vi "GetEventHardpointMonitorWarningField.vi"(10 "Event Data":string, 11 "Cluster in":refnum<vi>) -> (3 "Array":string[](array[string]))   [LabVIEW 2016]
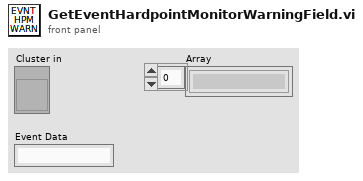
[diagram p1: front panel]
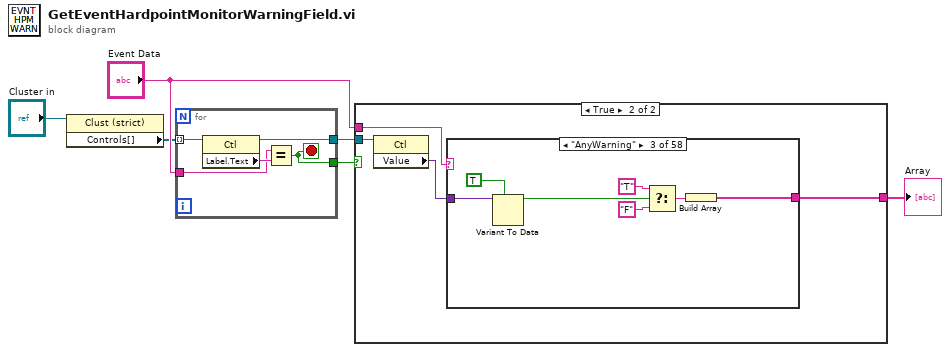
[diagram p0: block diagram]
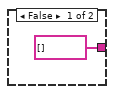
[diagram p2: hidden frame]
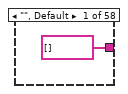
[diagram p3: hidden frame]
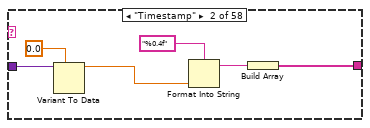
[diagram p4: hidden frame]
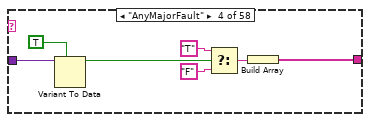
[diagram p5: hidden frame]
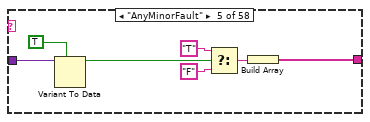
[diagram p6: hidden frame]
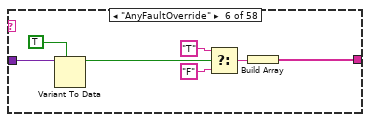
[diagram p7: hidden frame]
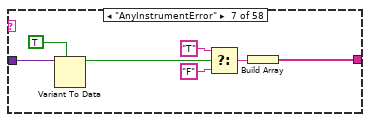
[diagram p8: hidden frame]
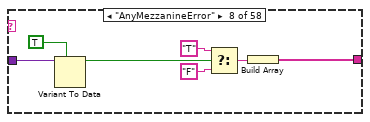
[diagram p9: hidden frame]
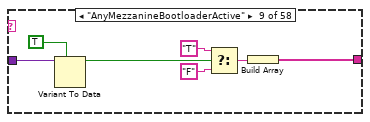
[diagram p10: hidden frame]
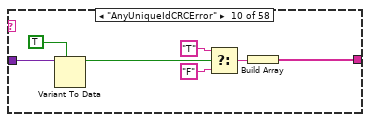
[diagram p11: hidden frame]
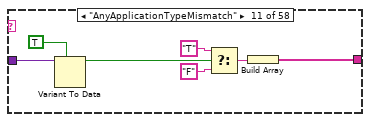
[diagram p12: hidden frame]
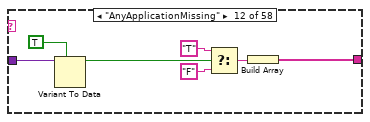
[diagram p13: hidden frame]
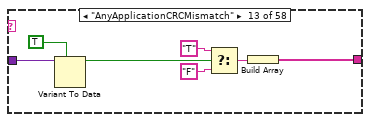
[diagram p14: hidden frame]
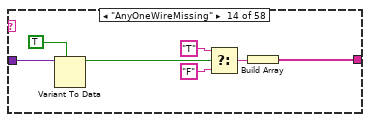
[diagram p15: hidden frame]
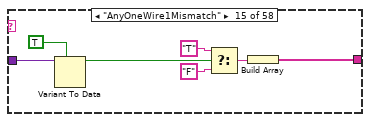
[diagram p16: hidden frame]
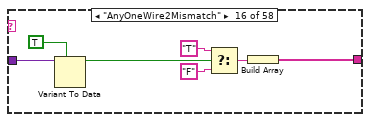
[diagram p17: hidden frame]
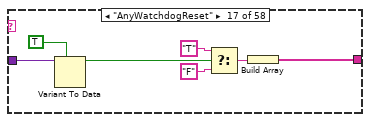
[diagram p18: hidden frame]
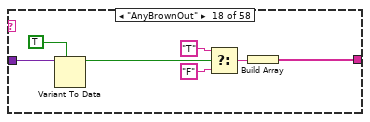
[diagram p19: hidden frame]
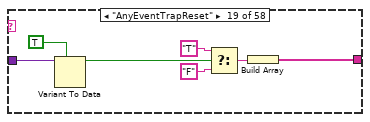
[diagram p20: hidden frame]
diagram:
  n1 = property on="Property Node" class="Clust (strict)"(reference="Cluster in") -> ("Controls[]"=w3:refnum<vi>[])  [unwired: 1 in, 2 out]
  n2 = for {
    tunnel: w3 -> [w11] mode=indexing
    tunnel: [w10] -> w5
    tunnel: "Event Data" -> [w8]
    tunnel: [w7] -> w6
    stop <- w7 stop-if-true
    n3 = property on="Property Node" class="Ctl"(reference=w11) -> (reference out=w10:refnum<vi>, "Label.Text"=w9:string)  [unwired: 1 in, 1 out]
    n4 = Equal?(x=w8, y=w9) -> (x = y?=w7:bool)
  }
  n5 = case shown="True" w6 {
    tunnel: "Event Data" -> [_ w16]
    tunnel: w5 -> [_ w15]
    tunnel: [string[] [] w13] -> w2
    frame False {
    }
    frame True {
      n6 = property on="Property Node" class="Ctl"(reference=w15) -> ("Value"=w14:variant)  [unwired: 1 in, 2 out]
      n7 = case shown="\"AnyWarning\"" w16 {
        tunnel: [string[] [] w21 w24 w31 w38 w45 w52 w59 w66 w73 w80 w87 w94 w101 w108 w115 w122 w129 w136 w143 w150 w157 w164 w171 w178 w185 w192 w199 w206 w213 w220 w228 w236 w244 w252 w260 w268 w276 w284 w292 w300 w308 w316 w324 w332 w340 w348 w356 w364 w372 w380 w388 w396 w404 w412 w420 w428 w439] -> w13
        tunnel: w14 -> [_ w19 w30 w37 w44 w51 w58 w65 w72 w79 w86 w93 w100 w107 w114 w121 w128 w135 w142 w149 w156 w163 w170 w177 w184 w191 w198 w205 w212 w219 w223 w231 w239 w247 w255 w263 w271 w279 w287 w295 w303 w311 w319 w327 w335 w343 w351 w359 w367 w375 w383 w391 w399 w407 w415 w423 w431 w437]
        frame "", Default {
        }
        frame "Timestamp" {
          n8 = Variant To Data(type=0.0, Variant=w19) -> (data=w20:dbl)  [unwired: 1 in, 1 out]
          n9 = Format Into String(format string="%0.4f", w20) -> (resulting string=w22:string)  [unwired: 2 in, 1 out]
          n10 = Build Array(w22) -> (w21:string[])
        }
        frame "AnyWarning" {
          n11 = Variant To Data(type=TRUE, Variant=w30) -> (data=w28:bool)  [unwired: 1 in, 1 out]
          n12 = Select(t="T", s=w28, f="F") -> (s? t:f=w25:string)
          n13 = Build Array(w25) -> (w24:string[])
        }
        frame "AnyMajorFault" {
          n14 = Variant To Data(type=TRUE, Variant=w37) -> (data=w35:bool)  [unwired: 1 in, 1 out]
          n15 = Select(t="T", s=w35, f="F") -> (s? t:f=w32:string)
          n16 = Build Array(w32) -> (w31:string[])
        }
        frame "AnyMinorFault" {
          n17 = Variant To Data(type=TRUE, Variant=w44) -> (data=w42:bool)  [unwired: 1 in, 1 out]
          n18 = Select(t="T", s=w42, f="F") -> (s? t:f=w39:string)
          n19 = Build Array(w39) -> (w38:string[])
        }
        frame "AnyFaultOverride" {
          n20 = Variant To Data(type=TRUE, Variant=w51) -> (data=w49:bool)  [unwired: 1 in, 1 out]
          n21 = Select(t="T", s=w49, f="F") -> (s? t:f=w46:string)
          n22 = Build Array(w46) -> (w45:string[])
        }
        frame "AnyInstrumentError" {
          n23 = Variant To Data(type=TRUE, Variant=w58) -> (data=w56:bool)  [unwired: 1 in, 1 out]
          n24 = Select(t="T", s=w56, f="F") -> (s? t:f=w53:string)
          n25 = Build Array(w53) -> (w52:string[])
        }
        frame "AnyMezzanineError" {
          n26 = Variant To Data(type=TRUE, Variant=w65) -> (data=w63:bool)  [unwired: 1 in, 1 out]
          n27 = Select(t="T", s=w63, f="F") -> (s? t:f=w60:string)
          n28 = Build Array(w60) -> (w59:string[])
        }
        frame "AnyMezzanineBootloaderActive" {
          n29 = Variant To Data(type=TRUE, Variant=w72) -> (data=w70:bool)  [unwired: 1 in, 1 out]
          n30 = Select(t="T", s=w70, f="F") -> (s? t:f=w67:string)
          n31 = Build Array(w67) -> (w66:string[])
        }
        frame "AnyUniqueIdCRCError" {
          n32 = Variant To Data(type=TRUE, Variant=w79) -> (data=w77:bool)  [unwired: 1 in, 1 out]
          n33 = Select(t="T", s=w77, f="F") -> (s? t:f=w74:string)
          n34 = Build Array(w74) -> (w73:string[])
        }
        frame "AnyApplicationTypeMismatch" {
          n35 = Variant To Data(type=TRUE, Variant=w86) -> (data=w84:bool)  [unwired: 1 in, 1 out]
          n36 = Select(t="T", s=w84, f="F") -> (s? t:f=w81:string)
          n37 = Build Array(w81) -> (w80:string[])
        }
        frame "AnyApplicationMissing" {
          n38 = Variant To Data(type=TRUE, Variant=w93) -> (data=w91:bool)  [unwired: 1 in, 1 out]
          n39 = Select(t="T", s=w91, f="F") -> (s? t:f=w88:string)
          n40 = Build Array(w88) -> (w87:string[])
        }
        frame "AnyApplicationCRCMismatch" {
          n41 = Variant To Data(type=TRUE, Variant=w100) -> (data=w98:bool)  [unwired: 1 in, 1 out]
          n42 = Select(t="T", s=w98, f="F") -> (s? t:f=w95:string)
          n43 = Build Array(w95) -> (w94:string[])
        }
        frame "AnyOneWireMissing" {
          n44 = Variant To Data(type=TRUE, Variant=w107) -> (data=w105:bool)  [unwired: 1 in, 1 out]
          n45 = Select(t="T", s=w105, f="F") -> (s? t:f=w102:string)
          n46 = Build Array(w102) -> (w101:string[])
        }
        frame "AnyOneWire1Mismatch" {
          n47 = Variant To Data(type=TRUE, Variant=w114) -> (data=w112:bool)  [unwired: 1 in, 1 out]
          n48 = Select(t="T", s=w112, f="F") -> (s? t:f=w109:string)
          n49 = Build Array(w109) -> (w108:string[])
        }
        frame "AnyOneWire2Mismatch" {
          n50 = Variant To Data(type=TRUE, Variant=w121) -> (data=w119:bool)  [unwired: 1 in, 1 out]
          n51 = Select(t="T", s=w119, f="F") -> (s? t:f=w116:string)
          n52 = Build Array(w116) -> (w115:string[])
        }
        frame "AnyWatchdogReset" {
          n53 = Variant To Data(type=TRUE, Variant=w128) -> (data=w126:bool)  [unwired: 1 in, 1 out]
          n54 = Select(t="T", s=w126, f="F") -> (s? t:f=w123:string)
          n55 = Build Array(w123) -> (w122:string[])
        }
        frame "AnyBrownOut" {
          n56 = Variant To Data(type=TRUE, Variant=w135) -> (data=w133:bool)  [unwired: 1 in, 1 out]
          n57 = Select(t="T", s=w133, f="F") -> (s? t:f=w130:string)
          n58 = Build Array(w130) -> (w129:string[])
        }
        frame "AnyEventTrapReset" {
          n59 = Variant To Data(type=TRUE, Variant=w142) -> (data=w140:bool)  [unwired: 1 in, 1 out]
          n60 = Select(t="T", s=w140, f="F") -> (s? t:f=w137:string)
          n61 = Build Array(w137) -> (w136:string[])
        }
        frame "AnySSRPowerFault" {
          n62 = Variant To Data(type=TRUE, Variant=w149) -> (data=w147:bool)  [unwired: 1 in, 1 out]
          n63 = Select(t="T", s=w147, f="F") -> (s? t:f=w144:string)
          n64 = Build Array(w144) -> (w143:string[])
        }
        frame "AnyAuxPowerFault" {
          n65 = Variant To Data(type=TRUE, Variant=w156) -> (data=w154:bool)  [unwired: 1 in, 1 out]
          n66 = Select(t="T", s=w154, f="F") -> (s? t:f=w151:string)
          n67 = Build Array(w151) -> (w150:string[])
        }
        frame "AnyMezzanineS1AInterface1Fault" {
          n68 = Variant To Data(type=TRUE, Variant=w163) -> (data=w161:bool)  [unwired: 1 in, 1 out]
          n69 = Select(t="T", s=w161, f="F") -> (s? t:f=w158:string)
          n70 = Build Array(w158) -> (w157:string[])
        }
        frame "AnyMezzanineS1ALVDT1Fault" {
          n71 = Variant To Data(type=TRUE, Variant=w170) -> (data=w168:bool)  [unwired: 1 in, 1 out]
          n72 = Select(t="T", s=w168, f="F") -> (s? t:f=w165:string)
          n73 = Build Array(w165) -> (w164:string[])
        }
        frame "AnyMezzanineS1AInterface2Fault" {
          n74 = Variant To Data(type=TRUE, Variant=w177) -> (data=w175:bool)  [unwired: 1 in, 1 out]
          n75 = Select(t="T", s=w175, f="F") -> (s? t:f=w172:string)
          n76 = Build Array(w172) -> (w171:string[])
        }
        frame "AnyMezzanineS1ALVDT2Fault" {
          n77 = Variant To Data(type=TRUE, Variant=w184) -> (data=w182:bool)  [unwired: 1 in, 1 out]
          n78 = Select(t="T", s=w182, f="F") -> (s? t:f=w179:string)
          n79 = Build Array(w179) -> (w178:string[])
        }
        frame "AnyMezzanineUniqueIdCRCError" {
          n80 = Variant To Data(type=TRUE, Variant=w191) -> (data=w189:bool)  [unwired: 1 in, 1 out]
          n81 = Select(t="T", s=w189, f="F") -> (s? t:f=w186:string)
          n82 = Build Array(w186) -> (w185:string[])
        }
        frame "AnyMezzanineEventTrapReset" {
          n83 = Variant To Data(type=TRUE, Variant=w198) -> (data=w196:bool)  [unwired: 1 in, 1 out]
          n84 = Select(t="T", s=w196, f="F") -> (s? t:f=w193:string)
          n85 = Build Array(w193) -> (w192:string[])
        }
        frame "AnyMezzanineDCPRS422ChipFault" {
          n86 = Variant To Data(type=TRUE, Variant=w205) -> (data=w203:bool)  [unwired: 1 in, 1 out]
          n87 = Select(t="T", s=w203, f="F") -> (s? t:f=w200:string)
          n88 = Build Array(w200) -> (w199:string[])
        }
        frame "AnyMezzanineApplicationMissing" {
          n89 = Variant To Data(type=TRUE, Variant=w212) -> (data=w210:bool)  [unwired: 1 in, 1 out]
          n90 = Select(t="T", s=w210, f="F") -> (s? t:f=w207:string)
          n91 = Build Array(w207) -> (w206:string[])
        }
        frame "AnyMezzanineApplicationCRCMismatch" {
          n92 = Variant To Data(type=TRUE, Variant=w219) -> (data=w217:bool)  [unwired: 1 in, 1 out]
          n93 = Select(t="T", s=w217, f="F") -> (s? t:f=w214:string)
          n94 = Build Array(w214) -> (w213:string[])
        }
        frame "MajorFault[6]" {
          n95 = Variant To Data(type=bool[] [], Variant=w223) -> (data=w221:bool[])  [unwired: 1 in, 1 out]
          n96 = for {
            tunnel: w221 -> [w227] mode=indexing
            tunnel: [w224] -> w220 mode=indexing
            n97 = Select(t="T", s=w227, f="F") -> (s? t:f=w224:string)
          }
        }
        frame "MinorFault[6]" {
          n98 = Variant To Data(type=bool[] [], Variant=w231) -> (data=w229:bool[])  [unwired: 1 in, 1 out]
          n99 = for {
            tunnel: w229 -> [w235] mode=indexing
            tunnel: [w232] -> w228 mode=indexing
            n100 = Select(t="T", s=w235, f="F") -> (s? t:f=w232:string)
          }
        }
        frame "FaultOverride[6]" {
          n101 = Variant To Data(type=bool[] [], Variant=w239) -> (data=w237:bool[])  [unwired: 1 in, 1 out]
          n102 = for {
            tunnel: w237 -> [w243] mode=indexing
            tunnel: [w240] -> w236 mode=indexing
            n103 = Select(t="T", s=w243, f="F") -> (s? t:f=w240:string)
          }
        }
        frame "InstrumentError[6]" {
          n104 = Variant To Data(type=bool[] [], Variant=w247) -> (data=w245:bool[])  [unwired: 1 in, 1 out]
          n105 = for {
            tunnel: w245 -> [w251] mode=indexing
            tunnel: [w248] -> w244 mode=indexing
            n106 = Select(t="T", s=w251, f="F") -> (s? t:f=w248:string)
          }
        }
        frame "MezzanineError[6]" {
          n107 = Variant To Data(type=bool[] [], Variant=w255) -> (data=w253:bool[])  [unwired: 1 in, 1 out]
          n108 = for {
            tunnel: w253 -> [w259] mode=indexing
            tunnel: [w256] -> w252 mode=indexing
            n109 = Select(t="T", s=w259, f="F") -> (s? t:f=w256:string)
          }
        }
        frame "MezzanineBootloaderActive[6]" {
          n110 = Variant To Data(type=bool[] [], Variant=w263) -> (data=w261:bool[])  [unwired: 1 in, 1 out]
          n111 = for {
            tunnel: w261 -> [w267] mode=indexing
            tunnel: [w264] -> w260 mode=indexing
            n112 = Select(t="T", s=w267, f="F") -> (s? t:f=w264:string)
          }
        }
        frame "UniqueIdCRCError[6]" {
          n113 = Variant To Data(type=bool[] [], Variant=w271) -> (data=w269:bool[])  [unwired: 1 in, 1 out]
          n114 = for {
            tunnel: w269 -> [w275] mode=indexing
            tunnel: [w272] -> w268 mode=indexing
            n115 = Select(t="T", s=w275, f="F") -> (s? t:f=w272:string)
          }
        }
        frame "ApplicationTypeMismatch[6]" {
          n116 = Variant To Data(type=bool[] [], Variant=w279) -> (data=w277:bool[])  [unwired: 1 in, 1 out]
          n117 = for {
            tunnel: w277 -> [w283] mode=indexing
            tunnel: [w280] -> w276 mode=indexing
            n118 = Select(t="T", s=w283, f="F") -> (s? t:f=w280:string)
          }
        }
        frame "ApplicationMissing[6]" {
          n119 = Variant To Data(type=bool[] [], Variant=w287) -> (data=w285:bool[])  [unwired: 1 in, 1 out]
          n120 = for {
            tunnel: w285 -> [w291] mode=indexing
            tunnel: [w288] -> w284 mode=indexing
            n121 = Select(t="T", s=w291, f="F") -> (s? t:f=w288:string)
          }
        }
        frame "ApplicationCRCMismatch[6]" {
          n122 = Variant To Data(type=bool[] [], Variant=w295) -> (data=w293:bool[])  [unwired: 1 in, 1 out]
          n123 = for {
            tunnel: w293 -> [w299] mode=indexing
            tunnel: [w296] -> w292 mode=indexing
            n124 = Select(t="T", s=w299, f="F") -> (s? t:f=w296:string)
          }
        }
        frame "OneWireMissing[6]" {
          n125 = Variant To Data(type=bool[] [], Variant=w303) -> (data=w301:bool[])  [unwired: 1 in, 1 out]
          n126 = for {
            tunnel: w301 -> [w307] mode=indexing
            tunnel: [w304] -> w300 mode=indexing
            n127 = Select(t="T", s=w307, f="F") -> (s? t:f=w304:string)
          }
        }
        frame "OneWire1Mismatch[6]" {
          n128 = Variant To Data(type=bool[] [], Variant=w311) -> (data=w309:bool[])  [unwired: 1 in, 1 out]
          n129 = for {
            tunnel: w309 -> [w315] mode=indexing
            tunnel: [w312] -> w308 mode=indexing
            n130 = Select(t="T", s=w315, f="F") -> (s? t:f=w312:string)
          }
        }
        frame "OneWire2Mismatch[6]" {
          n131 = Variant To Data(type=bool[] [], Variant=w319) -> (data=w317:bool[])  [unwired: 1 in, 1 out]
          n132 = for {
            tunnel: w317 -> [w323] mode=indexing
            tunnel: [w320] -> w316 mode=indexing
            n133 = Select(t="T", s=w323, f="F") -> (s? t:f=w320:string)
          }
        }
        frame "WatchdogReset[6]" {
          n134 = Variant To Data(type=bool[] [], Variant=w327) -> (data=w325:bool[])  [unwired: 1 in, 1 out]
          n135 = for {
            tunnel: w325 -> [w331] mode=indexing
            tunnel: [w328] -> w324 mode=indexing
            n136 = Select(t="T", s=w331, f="F") -> (s? t:f=w328:string)
          }
        }
        frame "BrownOut[6]" {
          n137 = Variant To Data(type=bool[] [], Variant=w335) -> (data=w333:bool[])  [unwired: 1 in, 1 out]
          n138 = for {
            tunnel: w333 -> [w339] mode=indexing
            tunnel: [w336] -> w332 mode=indexing
            n139 = Select(t="T", s=w339, f="F") -> (s? t:f=w336:string)
          }
        }
        frame "EventTrapReset[6]" {
          n140 = Variant To Data(type=bool[] [], Variant=w343) -> (data=w341:bool[])  [unwired: 1 in, 1 out]
          n141 = for {
            tunnel: w341 -> [w347] mode=indexing
            tunnel: [w344] -> w340 mode=indexing
            n142 = Select(t="T", s=w347, f="F") -> (s? t:f=w344:string)
          }
        }
        frame "SSRPowerFault[6]" {
          n143 = Variant To Data(type=bool[] [], Variant=w351) -> (data=w349:bool[])  [unwired: 1 in, 1 out]
          n144 = for {
            tunnel: w349 -> [w355] mode=indexing
            tunnel: [w352] -> w348 mode=indexing
            n145 = Select(t="T", s=w355, f="F") -> (s? t:f=w352:string)
          }
        }
        frame "AuxPowerFault[6]" {
          n146 = Variant To Data(type=bool[] [], Variant=w359) -> (data=w357:bool[])  [unwired: 1 in, 1 out]
          n147 = for {
            tunnel: w357 -> [w363] mode=indexing
            tunnel: [w360] -> w356 mode=indexing
            n148 = Select(t="T", s=w363, f="F") -> (s? t:f=w360:string)
          }
        }
        frame "MezzanineS1AInterfaceFault[6]" {
          n149 = Variant To Data(type=bool[] [], Variant=w367) -> (data=w365:bool[])  [unwired: 1 in, 1 out]
          n150 = for {
            tunnel: w365 -> [w371] mode=indexing
            tunnel: [w368] -> w364 mode=indexing
            n151 = Select(t="T", s=w371, f="F") -> (s? t:f=w368:string)
          }
        }
        frame "MezzanineS1ALVDT1Fault[6]" {
          n152 = Variant To Data(type=bool[] [], Variant=w375) -> (data=w373:bool[])  [unwired: 1 in, 1 out]
          n153 = for {
            tunnel: w373 -> [w379] mode=indexing
            tunnel: [w376] -> w372 mode=indexing
            n154 = Select(t="T", s=w379, f="F") -> (s? t:f=w376:string)
          }
        }
        frame "MezzanineS1AInterface2Fault[6]" {
          n155 = Variant To Data(type=bool[] [], Variant=w383) -> (data=w381:bool[])  [unwired: 1 in, 1 out]
          n156 = for {
            tunnel: w381 -> [w387] mode=indexing
            tunnel: [w384] -> w380 mode=indexing
            n157 = Select(t="T", s=w387, f="F") -> (s? t:f=w384:string)
          }
        }
        frame "MezzanineS1ALVDT2Fault[6]" {
          n158 = Variant To Data(type=bool[] [], Variant=w391) -> (data=w389:bool[])  [unwired: 1 in, 1 out]
          n159 = for {
            tunnel: w389 -> [w395] mode=indexing
            tunnel: [w392] -> w388 mode=indexing
            n160 = Select(t="T", s=w395, f="F") -> (s? t:f=w392:string)
          }
        }
        frame "MezzanineUniqueIdCRCError[6]" {
          n161 = Variant To Data(type=bool[] [], Variant=w399) -> (data=w397:bool[])  [unwired: 1 in, 1 out]
          n162 = for {
            tunnel: w397 -> [w403] mode=indexing
            tunnel: [w400] -> w396 mode=indexing
            n163 = Select(t="T", s=w403, f="F") -> (s? t:f=w400:string)
          }
        }
        frame "MezzanineEventTrapReset[6]" {
          n164 = Variant To Data(type=bool[] [], Variant=w407) -> (data=w405:bool[])  [unwired: 1 in, 1 out]
          n165 = for {
            tunnel: w405 -> [w411] mode=indexing
            tunnel: [w408] -> w404 mode=indexing
            n166 = Select(t="T", s=w411, f="F") -> (s? t:f=w408:string)
          }
        }
        frame "MezzanineDCPRS422ChipFault[6]" {
          n167 = Variant To Data(type=bool[] [], Variant=w415) -> (data=w413:bool[])  [unwired: 1 in, 1 out]
          n168 = for {
            tunnel: w413 -> [w419] mode=indexing
            tunnel: [w416] -> w412 mode=indexing
            n169 = Select(t="T", s=w419, f="F") -> (s? t:f=w416:string)
          }
        }
        frame "MezzanineApplicationMissing[6]" {
          n170 = Variant To Data(type=bool[] [], Variant=w423) -> (data=w421:bool[])  [unwired: 1 in, 1 out]
          n171 = for {
            tunnel: w421 -> [w427] mode=indexing
            tunnel: [w424] -> w420 mode=indexing
            n172 = Select(t="T", s=w427, f="F") -> (s? t:f=w424:string)
          }
        }
        frame "MezzanineApplicationCRCMismatch[6]" {
          n173 = Variant To Data(type=bool[] [], Variant=w431) -> (data=w429:bool[])  [unwired: 1 in, 1 out]
          n174 = for {
            tunnel: w429 -> [w435] mode=indexing
            tunnel: [w432] -> w428 mode=indexing
            n175 = Select(t="T", s=w435, f="F") -> (s? t:f=w432:string)
          }
        }
        frame "priority" {
          n176 = Variant To Data(type=0, Variant=w437) -> (data=w438:i32)  [unwired: 1 in, 1 out]
          n177 = Format Into String(format string="%d", w438) -> (resulting string=w440:string)  [unwired: 2 in, 1 out]
          n178 = Build Array(w440) -> (w439:string[])
        }
      }
    }
  }
  "Array" <- w2
